vi "State_Machine.vi"(8 "error in (no error)":errorcluster caption="entrée d'erreur (pas d'erreur)", 11 "Get_Voltage en entrée":refnum<class "Zigbee_Extpanid.lvclass">) -> (0 "error out":errorcluster caption="sortie d'erreur", 2 "Json_String":string, 3 "Get_Voltage en sortie":refnum<class "Zigbee_Extpanid.lvclass">)   [LabVIEW 2020, in "Library Test.lvlib" / "Zigbee_Extpanid.lvclass"]
uses:
  Zigbee_Extpanid.lvclass
  C:/Users/ngarcin/OneDrive - Altyor/Standard TB/Class/Test/Test (Default)/Test (Default).lvclass
  C:/Users/ngarcin/OneDrive - Altyor/Standard TB/Class/Test/Zigbee_Send_Command_UART/Zigbee_Send_Command_UART.lvclass
  JSON API/JSON Value/Set from JSON string.vi
  JSON API/JSON Value/JSON Value.lvclass
  Zigbee_Send_Command_UART/Zigbee_Send_Command_UART.lvclass
  Zigbee_Extpanid.lvclass/Zigbee_Extpanid.ctl
  JSON API/Variant JSON/Variant JSON.lvlib
  JSON API/Get Polymorphic/JSON GetSet.lvlib
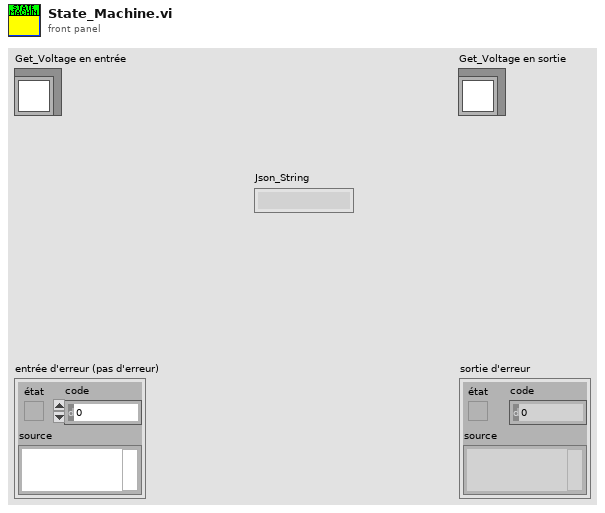
[diagram p1: front panel]
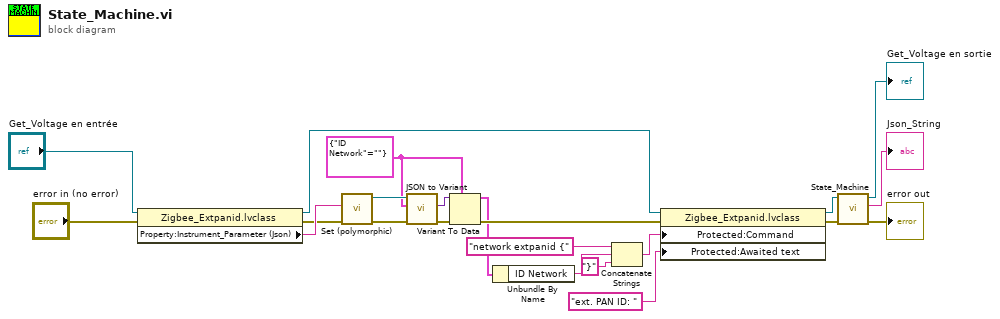
[diagram p0: block diagram]
diagram:
  w13 = cluster{"ID Network":string} {"ID Network"=""}
  n1 = property class="Zigbee_Extpanid.lvclass"(reference="Get_Voltage en entrée", error in="error in (no error)") -> (reference out=w11:refnum<class "Zigbee_Extpanid.lvclass">, error out=w14:errorcluster, "Property:Instrument_Parameter (Json)"=w15:string)
  n2 = call-poly "Set (polymorphic).vi"("error in (no error)"=w14, "JSON stream"=w15) -> ("error out"=w17:errorcluster, "JSON Value out"=w19:refnum<class "JSON Value.lvclass">)  [unwired: 7 in, 1 out]
  n3 = call "JSON to Variant.vi"("error in (no error)"=w17, "Variant (Data Type)"=w13, "JSON Value"=w19) -> ("error out"=w18:errorcluster, "Variant out"=w16:variant)  [unwired: 7 in]
  n4 = Variant To Data(error in=w18, type=w13, Variant=w16) -> (data=w10:cluster{"ID Network":string}, error out=w12:errorcluster)
  n5 = Unbundle By Name(w10) -> ("ID Network"=w8:string)
  n6 = Concatenate Strings("network extpanid {" ("Command"), w8, "}" ("chaîne")) -> (w6:string)
  n7 = property class="Zigbee_Extpanid.lvclass"(reference=w11, error in=w12, "Protected:Command"=w6, "Protected:Awaited text"="ext. PAN ID: " ("Awaited text")) -> (reference out=w3:refnum<class "Zigbee_Extpanid.lvclass">, error out=w2:errorcluster)
  n8 = call-parent "State_Machine.vi"("error in (no error)"=w2, "Send_Frame en entrée"=w3) -> ("error out"=→"error out":errorcluster, "Json_String"=→"Json_String":string, "Send_Frame en sortie"=→"Get_Voltage en sortie":refnum<class "Zigbee_Extpanid.lvclass">)  [unwired: 7 in]
